vi "Add Profile to File.vi"(8 "error in":errorcluster, 10 "Profile":T1, 11 "File Path":path) -> (0 "error out":errorcluster)   [LabVIEW 2025, in "TS Environment Manager.lvlib"]
doc: "This VI adds a new profile to a configuration file if the profile name does not already exist. Also the version format is validated."
uses:
  TS Environment Manager.lvlib
  Type Definitions/Profile--cluster.ctl
  Type Definitions/Architecture--enum.ctl
  <vilib>/Utility/config.llb/Write Key (String).vi
  <vilib>/Utility/config.llb/Write Key (Path).vi
  <vilib>/regexp/Match Regular Expression.xnode
  <vilib>/Utility/config.llb/NI_LVConfig.lvlib
  <userlib>/_OpenG.lib/file/file.llb/openg_file.lvlib
  <userlib>/_OpenG.lib/file/file.llb/Strip Path Extension - Path__ogtk.vi
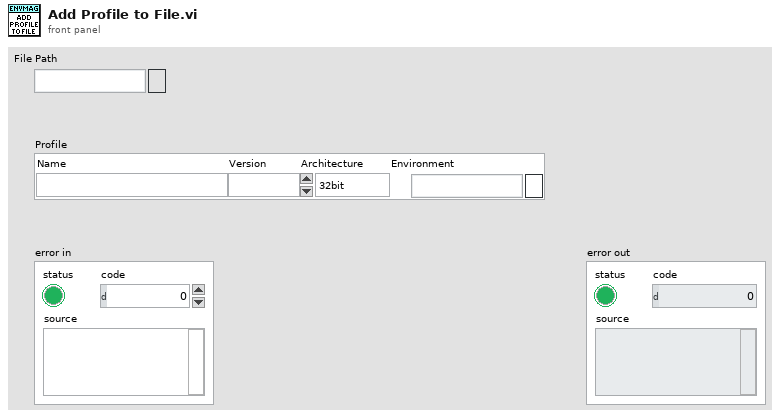
[diagram p1: front panel]
types:
  T1 = typedef "Profile--cluster.ctl" = cluster{"Name":string, "Version":string, "Architecture":T2, "Environment":path}
  T2 = typedef "Architecture--enum.ctl" = enum16{"32bit", "64bit"}
  T3 = typedef "NI_LVConfig.lvlib/Config Data RefNum.ctl" = refnum<k1>
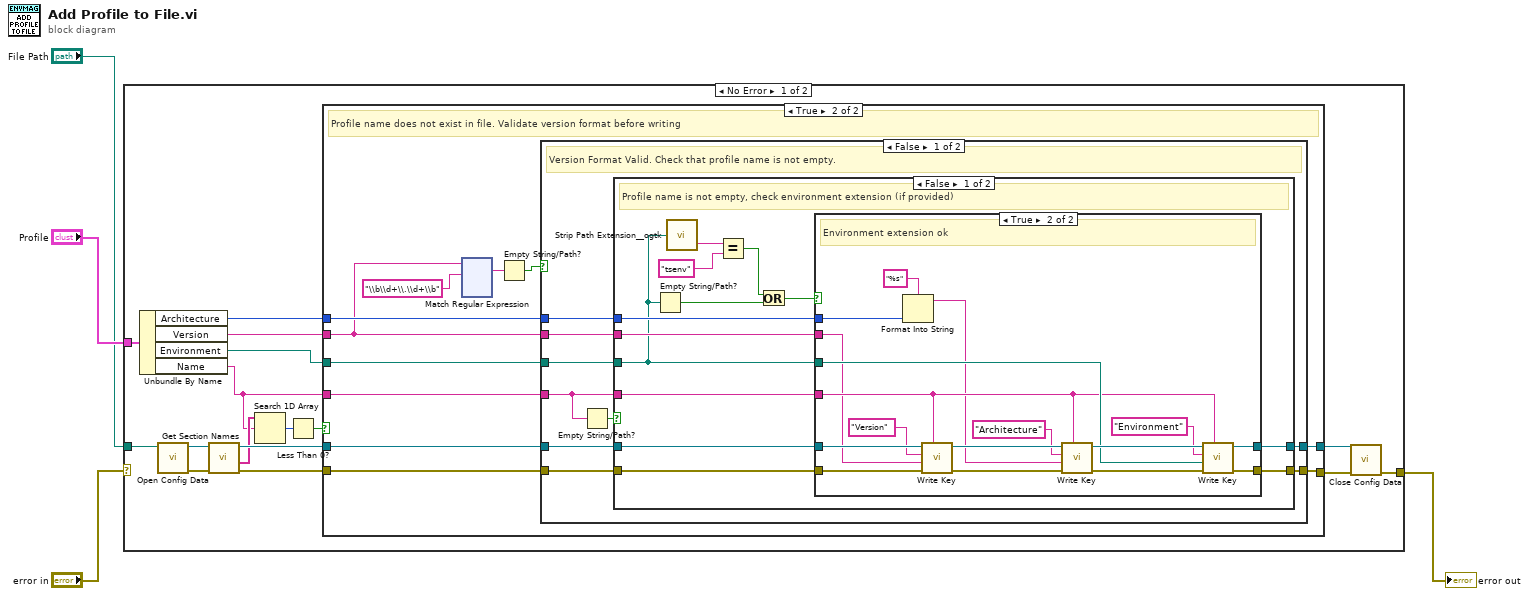
[diagram p0: block diagram]
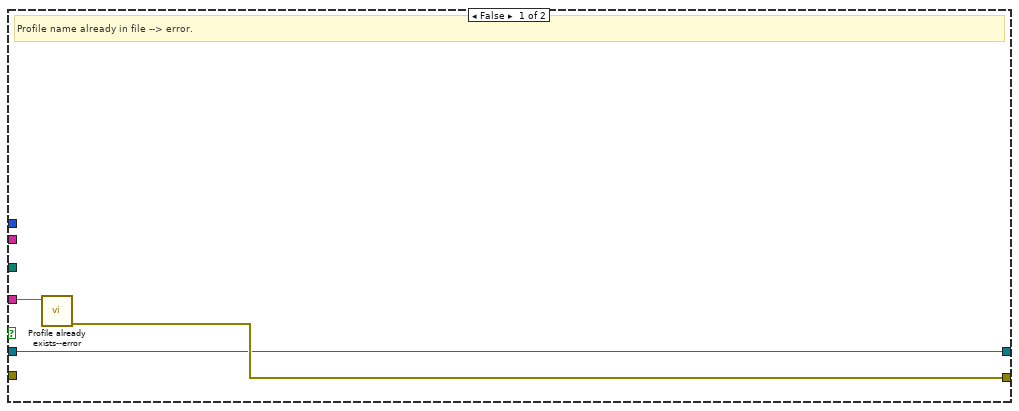
[diagram p2: hidden frame]
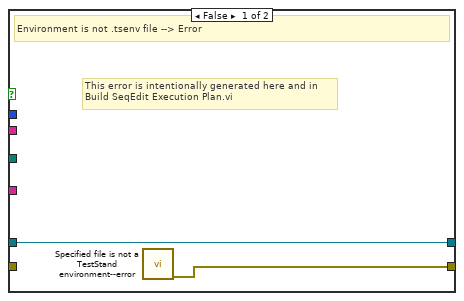
[diagram p3: hidden frame]
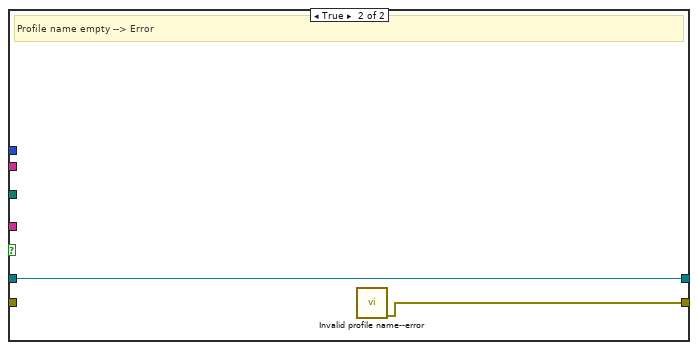
[diagram p4: hidden frame]
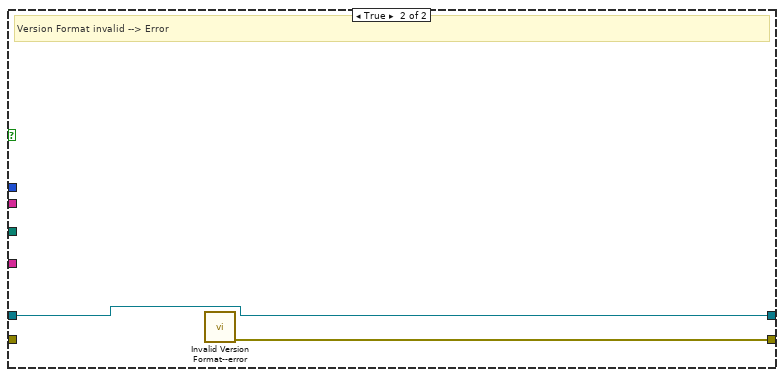
[diagram p5: hidden frame]
diagram:
  n1 = case shown="No Error" "error in" {
    selector: "error in" -> [_ w197]
    tunnel: "Profile" -> [w13 _]
    tunnel: [w18 w197] -> w4
    tunnel: "File Path" -> [w7 _]
    frame No Error {
      n2 = Unbundle By Name(w13) -> ("Architecture"=w14:T2, "Version"=w15:string, "Environment"=w16:path, "Name"=w5:string)
      n3 = call <vilib>:"Open Config Data.vi"("configuration file path"=w7) -> ("error out"=w19:errorcluster, "refnum"=w8:T3)  [unwired: 8 in, 1 out]
      n4 = call <vilib>:"Get Section Names.vi"("error in (no error)"=w19, "refnum"=w8) -> ("error out"=w20:errorcluster, "section names"=w9:string[], "refnum out"=w12:T3)  [unwired: 7 in]
      n5 = Search 1D Array(1D array=w9, element=w5) -> (index of element=w10:i32)  [unwired: 1 in]
      n6 = Less Than 0?(x=w10) -> (x < 0?=w11:bool)
      n7 = case shown="True" w11 {
        tunnel: w5 -> [w22 w29]
        tunnel: [w23 w33] -> w17
        tunnel: w12 -> [w21 w32]
        tunnel: w20 -> [_ w34]
        tunnel: w15 -> [_ w25]
        tunnel: w14 -> [_ w28]
        tunnel: w16 -> [_ w31]
        tunnel: [w21 w30] -> w6
        frame False {
          # "Profile name already in file --> error."
          n8 = call "Profile already exists--error.vi"("Name"=w22) -> ("error out"=w23:errorcluster)  [unwired: 10 in]
        }
        frame True {
          # "Profile name does not exist in file. Validate version format before writing"
          n9 = xnode "Match Regular Expression"("input string"=w25, "regular expression"="\\b\\d+\\.\\d+\\b") -> ("whole match"=w26:string)  [unwired: 4 in, 4 out]
          n10 = Empty String/Path?(string/path=w26) -> (empty?=w24:bool)
          n11 = case shown="False" w24 {
            tunnel: w34 -> [w43 _]
            tunnel: [w42 w79] -> w33
            tunnel: w32 -> [w41 w78]
            tunnel: w31 -> [w40 _]
            tunnel: [w39 w78] -> w30
            tunnel: w29 -> [w36 _]
            tunnel: w28 -> [w38 _]
            tunnel: w25 -> [w37 _]
            frame False {
              # "Version Format Valid. Check that profile name is not empty."
              n12 = Empty String/Path?(string/path=w36) -> (empty?=w35:bool)
              n13 = case shown="False" w35 {
                tunnel: w43 -> [w56 _]
                tunnel: [w55 w77] -> w42
                tunnel: w41 -> [w54 w76]
                tunnel: w40 -> [w49 _]
                tunnel: [w53 w76] -> w39
                tunnel: w36 -> [w52 _]
                tunnel: w38 -> [w51 _]
                tunnel: w37 -> [w50 _]
                frame False {
                  # "Profile name is not empty, check environment extension (if provided)"
                  n14 = Empty String/Path?(string/path=w49) -> (empty?=w45:bool)
                  n15 = call-poly <userlib>:"Strip Path Extension__ogtk.vi"("path"=w49) -> ("extension"=w48:string)  [unwired: 1 out]
                  n16 = Equal?(x=w48, y="tsenv") -> (x = y?=w46:bool)
                  n17 = Or(x=w46, y=w45) -> (x .or. y?=w44:bool)
                  n18 = case shown="True" w44 {
                    tunnel: w56 -> [_ w75]
                    tunnel: [w58 w72] -> w55
                    tunnel: w54 -> [w57 w71]
                    tunnel: w49 -> [_ w65]
                    tunnel: [w57 w64] -> w53
                    tunnel: w52 -> [_ w63]
                    tunnel: w51 -> [_ w62]
                    tunnel: w50 -> [_ w59]
                    frame False {
                      # "This error is intentionally generated here and in \nBuild SeqEdit Execution Plan.vi"
                      # "Environment is not .tsenv file --> Error"
                      n19 = call "Specified file is not a TestStand environment--error.vi"() -> ("error out"=w58:errorcluster)  [unwired: 11 in]
                    }
                    frame True {
                      # "Environment extension ok"
                      n20 = Format Into String(format string="%s", w62) -> (resulting string=w60:string)  [unwired: 2 in, 1 out]
                      n21 = call-poly <vilib>:"Write Key.vi"("section"=w63, "error in (no error)"=w75, "value"=w59, "key"="Version", "refnum"=w71) -> ("error out"=w74:errorcluster, "refnum out"=w69:T3)  [unwired: 4 in, 1 out]
                      n22 = call-poly <vilib>:"Write Key.vi"("section"=w63, "error in (no error)"=w74, "value"=w60, "key"="Architecture", "refnum"=w69) -> ("error out"=w73:errorcluster, "refnum out"=w67:T3)  [unwired: 4 in, 1 out]
                      n23 = call-poly <vilib>:"Write Key.vi"("section"=w63, "error in (no error)"=w73, "value"=w65, "key"="Environment" ("section"), "refnum"=w67) -> ("error out"=w72:errorcluster, "refnum out"=w64:T3)  [unwired: 4 in, 1 out]
                    }
                  }
                }
                frame True {
                  # "Profile name empty --> Error"
                  n24 = call "Invalid profile name--error.vi"() -> ("error out"=w77:errorcluster)  [unwired: 11 in]
                }
              }
            }
            frame True {
              # "Version Format invalid --> Error"
              n25 = call "Invalid Version Format--error.vi"() -> ("error out"=w79:errorcluster)  [unwired: 11 in]
            }
          }
        }
      }
      n26 = call <vilib>:"Close Config Data.vi"("error in (no error)"=w17, "refnum"=w6) -> ("error out"=w18:errorcluster)  [unwired: 8 in, 1 out]
    }
    frame Error {
      # "Pass error without further action"
    }
  }
  "error out" <- w4
